vi "querey source settings menu small.vi"(0 "Enable":bool=TRUE, 1 "subvi?":bool, 5 "error in (no error)":errorcluster) -> (14 "Output cluster":T1={"Integer Timestamp"=0, "Needle Voltage"=0.0, "Frequency"=1.0, "Width (ms) : 0.1 "=0.05, "Desired Amplitude (V)"=0.0, "Settings ID"="", "ID#"=0} {"Needle Voltage" min=0.0 max=10.0 step=0.01 format="%.2g"; "Desired Amplitude (V)" min=0.0 max=10.0 step=0.01 format="%5.2f"; "Width (ms) : 0.1" min=0.05 max=5.0 step=0.01 format="%6.2f"; "Frequency" min=1.0 max=100.0 step=0.01 format="%.1f"}, 15 "Cancel loading":bool caption="Cancel", 18 "OK":bool, 19 "error out":errorcluster)   [LabVIEW 2012]
doc: "Displays a standard dialog box that prompts users to enter information, such as a user name and password.\n--------------------\n\nThis Express VI is configured as follows:\n\nMessage to Display to the User:\nThe inputs are: \nNumber: Upper Timestamp Range\nNumber: Lower Timestamp Range\nNumber: Settings ID"
uses:
  <vilib>/Utility/miscctls.llb/LVPointTypeDef.ctl
  <vilib>/addons/database/Auxilliary.llb/DB Tools Cursor Type.ctl
  <vilib>/addons/database/Connection.llb/Conn Execute.vi
  <vilib>/addons/database/Recordset.llb/Rec Fetch Recordset Data (R).vi
  <vilib>/addons/database/Recordset.llb/Rec Destroy - Connection.vi
  <vilib>/addons/database/_DB Variant To Data/Database Variant To Data.xnode
  <vilib>/addons/database/NI_Database_API.lvlib
panel:
  in  "Tag Filter":string
  out "Settings":cluster{"String":string, "Value":dbl}[](array[cluster])
  in  "Settings ID Type":enum32{"All", "Saved", "Big Accel", "Automatic"}(radio)
  in  "Needle Voltage":dbl
  in  "Frequency":dbl
  in  "Width (ms) : 0.1":dbl
  in  "Desired Amplitude (V)":dbl
  out "Settings to be loaded":string
  in  "OK2":bool
  in  "Cancel":bool
  in  "Settings ID":i32(ring) items=["Any Settings ID."=-1, "Big Accelerator: olivine (saved at  1/29/2014 1:59:55 PM)"=6, "olivine (saved at  1/29/2014 1:54:08 PM)"=5, "Big Accelerator: olivine (saved at  1/29/2014 1:53:03 PM)"=4, "test (saved at  1/29/2014 1:49:37 PM)"=3, "Big Accelerator: test (saved at  1/29/2014 1:49:28 PM)"=2, "0"=1]
  in  "Lower Timestamp Range":timestamp
  in  "Upper Timestamp Range":timestamp
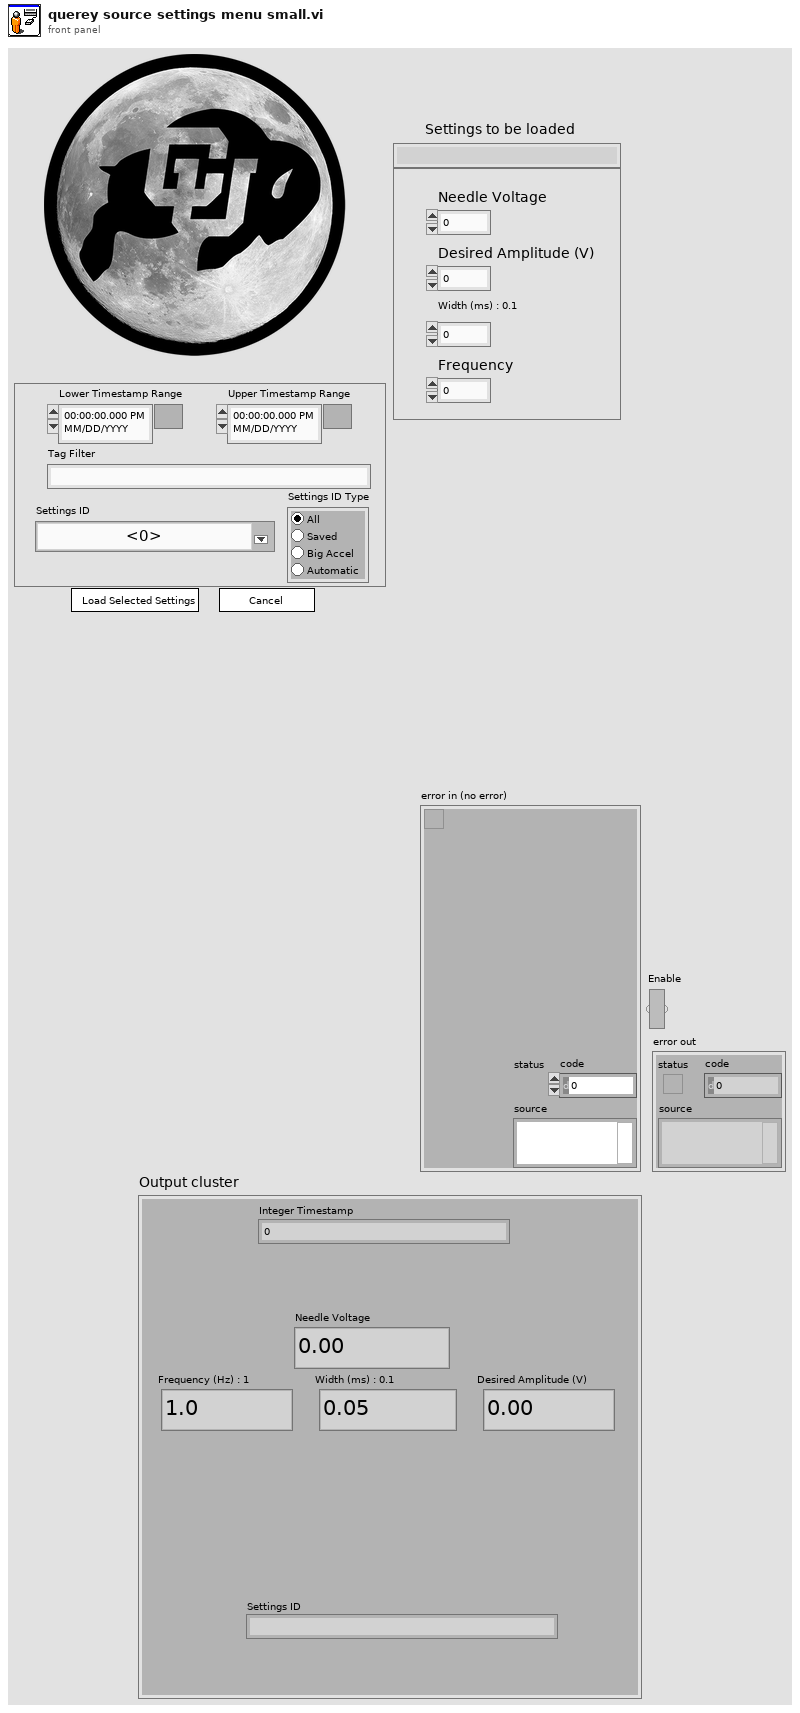
[diagram p1: front panel]
types:
  T1 = cluster{"Integer Timestamp":u64, "Needle Voltage":dbl, "Frequency":dbl, "Width (ms) : 0.1 ":dbl, "Desired Amplitude (V)":dbl, "Settings ID":string, "ID#":i32}
  T2 = typedef "LVPointTypeDef.ctl" = cluster{"Horizontal":i16, "Vertical":i16}
  T3 = enum32{"Invalid", "Standard", "Closed", "Hidden", "Minimized", "Maximized"}
  T4 = enum8{"Enabled", "Disabled", "Disabled and Grayed Out"}
  T5 = typedef "NI_Database_API.lvlib/DB Tools Cursor Type.ctl" = enum16{"forward-only", "keyset", "dynamic", "static"}
  T6 = typedef "NI_Database_API.lvlib/Conn ObjectReference.ctl" = refnum<k1>
  T7 = typedef "NI_Database_API.lvlib/Rec ObjectReference.ctl" = refnum<k1>
  T8 = typedef "dust_source_control_small.ctl" = cluster{"Integer Timestamp":u64, "Needle Voltage":dbl, "Frequency":dbl, "Width (ms) : 0.1 ":dbl, "Desired Amplitude (V)":dbl, "Settings ID":string, "ID#":i32}
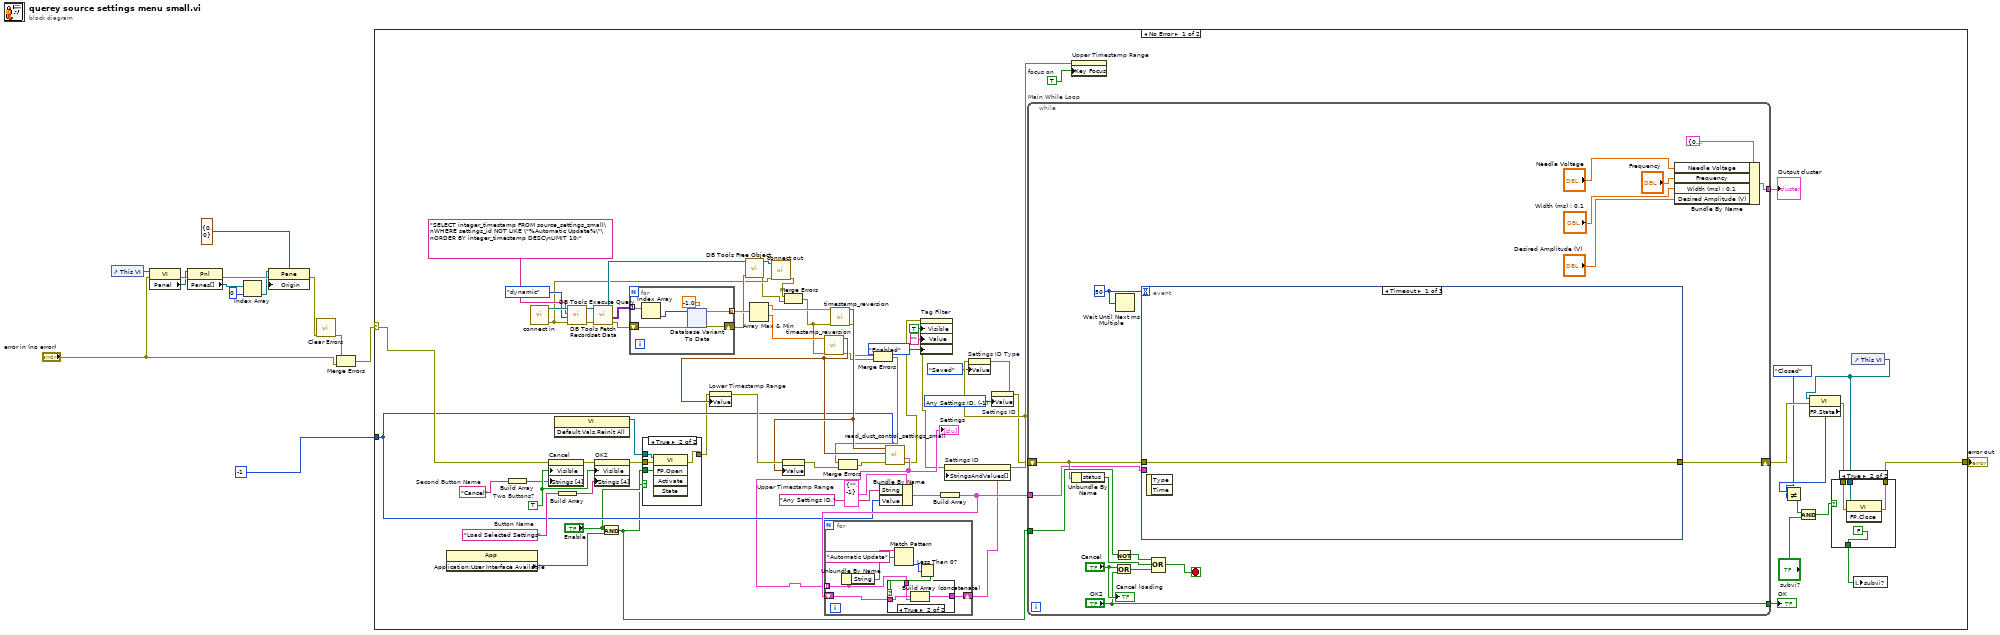
[diagram p0: block diagram]
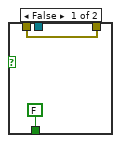
[diagram p2: hidden frame]
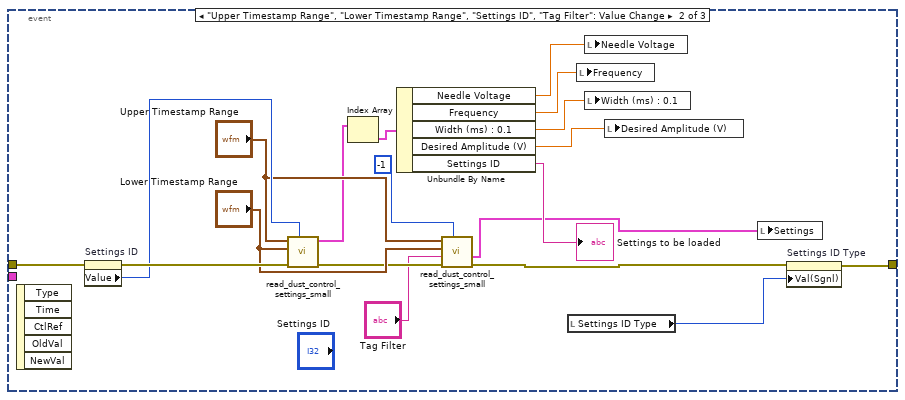
[diagram p5: hidden frame]
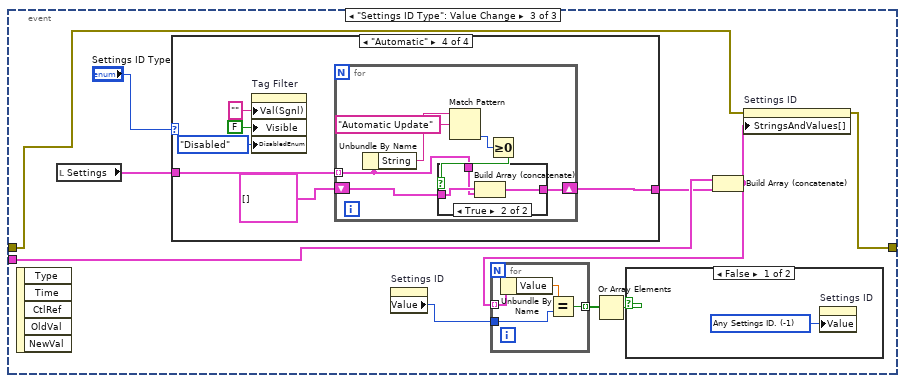
[diagram p6: hidden frame]
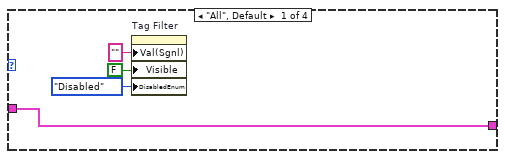
[diagram p8: hidden frame]
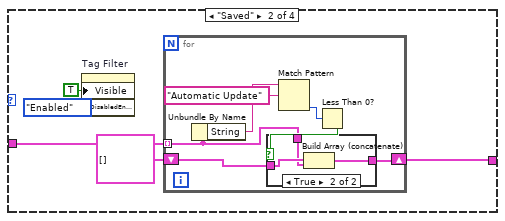
[diagram p9: hidden frame]
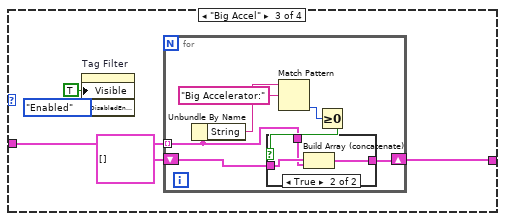
[diagram p11: hidden frame]
diagram:
  n1 = control-ref of="This VI"() -> (w12:refnum<vi>)
  n2 = property class="VI"(reference=w12, error in="error in (no error)") -> (error out=w11:errorcluster, "Panel"=w10:refnum<vi>)  [unwired: 1 out]
  n3 = property class="Pnl"(reference=w10, error in=w11) -> (error out=w9:errorcluster, "Panes[]"=w8:refnum<vi>[])  [unwired: 1 out]
  n4 = Index Array(array=w8, index=0) -> (element=w6:refnum<vi>)
  n5 = property class="Pane"(reference=w6, error in=w9, "Origin"=T2 {"Horizontal"=0, "Vertical"=0}) -> (error out=w4:errorcluster)  [unwired: 1 out]
  n6 = call <vilib>:"Clear Errors.vi"("error in (no error)"=w4) -> ("error out"=w2:errorcluster)  [unwired: 6 in]
  n7 = Merge Errors(w2, "error in (no error)") -> (w3:errorcluster)
  n8 = case shown="No Error" w3 {
    selector: w3 -> [w68 w248]
    tunnel: [w23 w248] -> w14
    tunnel: -1 ("Settings to be loaded") -> [w40 _]
    frame No Error {
      w35 = -1 items=["Any Settings ID."=-1, "Anna's Settings"=86, "Anna's Settings1"=87, "Test 'Test' \"Test\" test test."=97, "Test\""=91, "Test\""=92, "test 3"=82, "test 4"=83, "test mctesty"=88, "test mctesty"=89, "this is a \"test\" setting"=93] ("Settings ID")
      w74 = TRUE  # focus on
      w78 = "Cancel"  # Second Button Name
      w76 = "Load Selected Settings"  # Button Name
      w82 = TRUE  # Two Buttons?
      n9 = property class="App"() -> ("Application:User Interface Available"=w75:bool)  [unwired: 2 in, 2 out]
      n10 = Build Array(w78) -> (w79:string[])
      n11 = call "connect in.vi"() -> ("error out"=w52:errorcluster, "Database Connection"=w63:T6)  [unwired: 7 in, 1 out]
      n12 = property on="Cancel" class="Bool"(error in=w68, "Visible"=w82, "Strings [4]"=w79) -> (error out=w80:errorcluster)  [unwired: 1 in, 1 out]
      n13 = invoke class="VI" method="Default Vals.Reinit All"() -> (reference out=w29:refnum<vi>)  [unwired: 3 in, 2 out]
      n14 = Build Array(w76) -> (w77:string[])
      n15 = call-poly <vilib>:"DB Tools Execute Query.vi"("error in (no error)"=w52, "cursor type"=DB_Tools_Cursor_Type."dynamic", "SQL query"="SELECT integer_timestamp FROM source_settings_small\nWHERE settings_id NOT LIKE \"%Automatic Update%\"\nORDER BY integer_timestamp DESC\nLIMIT 10;" ("string"), "connection reference"=w63) -> ("error out"=w64:errorcluster, "recordset reference"=w65:T7)  [unwired: 4 in]
      n16 = call-poly <vilib>:"DB Tools Fetch Recordset Data.vi"("error in (no error)"=w64, "recordset reference"=w65) -> ("error out"=w59:errorcluster, "recordset data"=w60:variant[][], "recordset reference out"=w54:T7)  [unwired: 3 in]
      n17 = property on="OK2" class="Bool"(error in=w80, "Visible"=w82, "Strings [4]"=w77) -> (error out=w26:errorcluster)  [unwired: 1 in, 1 out]
      n18 = And(x="Enable", y=w75) -> (x .and. y?=w27:bool)
      n19 = for {
        tunnel: w60 -> [w109] mode=indexing
        tunnel: [w107] -> w58 mode=indexing
        shift-right: [w105] -> w53
        shift-left: w59 -> [w106]
        n20 = Index Array(array=w109) -> (element=w108:variant)  [unwired: 1 in]
        n21 = xnode "Database Variant To Data"("database variant"=w108, "error in (no error)"=w106, "type"=-1.0 ("Settings to be loaded")) -> ("data"=w107:dbl, "error out"=w105:errorcluster)
      }
      n22 = case shown="True" "Enable" {
        tunnel: w29 -> [_ w93]
        tunnel: w27 -> [_ w92]
        tunnel: w26 -> [w89 w91]
        tunnel: [w89 w90] -> w25
        frame False {
        }
        frame True {
          n23 = invoke class="VI" method="FP.Open"(reference=w93, error in=w91, "Activate"=w92) -> (error out=w90:errorcluster)  [unwired: 2 in, 4 out]
        }
      }
      n24 = call-poly <vilib>:"DB Tools Free Object.vi"("error in (no error)"=w53, "recordset reference"=w54) -> ("error out"=w51:errorcluster, "connection reference"=w55:T6)  [unwired: 8 in]
      n25 = Array Max & Min(array=w58) -> (max value=w57:dbl, min value=w56:dbl)  [unwired: 2 out]
      n26 = call "connect out.vi"("error in (no error)"=w52, "connection reference"=w55) -> ("error out"=w50:errorcluster)  [unwired: 9 in]
      n27 = Merge Errors(w50, w51) -> (w49:errorcluster)
      n28 = call "timestamp_reversion.vi"("error in (no error)"=w49, "Integer Timestamp"=w56) -> ("error out"=w45:errorcluster, "time stamp"=w47:timestamp)  [unwired: 7 in]
      n29 = property on="Lower Timestamp Range" class="AbsTime (strict)"(error in=w25, "Value"=w47) -> (error out=w72:errorcluster)  [unwired: 1 in, 1 out]
      n30 = call "timestamp_reversion.vi"("error in (no error)"=w49, "Integer Timestamp"=w57) -> ("error out"=w46:errorcluster, "time stamp"=w48:timestamp)  [unwired: 7 in]
      n31 = property on="Upper Timestamp Range" class="AbsTime (strict)"(error in=w72, "Value"=w48) -> (error out=w44:errorcluster)  [unwired: 1 in, 1 out]
      n32 = Merge Errors(w46, w45) -> (w43:errorcluster)
      n33 = Merge Errors(w43, w44) -> (w42:errorcluster)
      n34 = Bundle By Name(cluster=cluster{"String":string, "Value":i32} {"String"="", "Value"=-1}, "String"="Any Settings ID." ("Settings to be loaded"), "Value"=w40) -> (w69:cluster{"String":string, "Value":i32})
      n35 = call "read_dust_control_settings_small.vi"("Settings to be loaded"=w40, "error in (no error)"=w42, "Lower Timestamp Range"=w47, "Upper Timestamp Range"=w48) -> ("error out"=w32:errorcluster, "Array"=w38:cluster{"String":string, "Value":dbl}[])  [unwired: 5 in, 1 out]
      "Settings" <- w38
      n36 = property on="Tag Filter" class="Str"(error in=w32, "Visible"=TRUE, "Value"="" ("Tag"), "DisabledEnum"=T4."Enabled" ("Disabled")) -> (error out=w31:errorcluster)  [unwired: 1 in, 1 out]
      n37 = Build Array(w69) -> (w41:cluster{"String":string, "Value":i32}[])
      n38 = for {
        tunnel: w38 -> [w96] mode=indexing
        shift-right: [w95] -> w39
        shift-left: w41 -> [w97]
        n39 = Unbundle By Name(w96) -> ("String"=w100:string)
        n40 = Match Pattern(string=w100, regular expression="Automatic Update") -> (offset past match=w94:i32)  [unwired: 1 in, 3 out]
        n41 = Less Than 0?(x=w94) -> (x < 0?=w98:bool)
        n42 = case shown="True" w98 {
          tunnel: w97 -> [w101 w104]
          tunnel: w96 -> [_ w103]
          tunnel: [w101 w102] -> w95
          frame False {
          }
          frame True {
            n43 = Build Array (concatenate)(w104, w103) -> (w102:cluster{"String":string, "Value":dbl}[])
          }
        }
      }
      n44 = property on="Settings ID" class="Ring (strict)"(error in=w31, "StringsAndValues[]"=w39) -> (error out=w67:errorcluster)  [unwired: 1 in, 1 out]
      n45 = property on="Settings ID Type" class="RadioBtnsControl (strict)"(error in=w67, "Value"=enum32{"All", "Saved", "Big Accel", "Automatic"}."Saved" ("Settings ID Type")) -> (error out=w37:errorcluster)  [unwired: 1 in, 1 out]
      n46 = property on="Settings ID" class="Ring (strict)"(error in=w37, "Value"=w35) -> (error out=w36:errorcluster)  [unwired: 1 in, 1 out]
      n47 = while "Main While Loop" {
        tunnel: ["OK2"] -> w81
        tunnel: w27 -> [w158]
        tunnel: w41 -> [w143]
        tunnel: [w149] -> w73
        shift-right: [w151] -> w24
        shift-left: w36 -> [w152]
        stop <- w156 stop-if-true
        w150 = u32 50 ("millisecond multiple")
        n48 = Unbundle By Name(w152) -> ("status"=w154:bool)
        n49 = Or(x="Cancel", y="OK2") -> (x .or. y?=w155:bool)
        n50 = Not(x=w158) -> (.not. x?=w157:bool)
        n51 = Wait Until Next ms Multiple(millisecond multiple=w150) -> ()  [unwired: 1 out]
        n52 = event shown="[0] Timeout" {
          selector: _ -> [_ _ _]
          dyn-events: _ -> [_ _ _]
          timeout: w150 -> [_ _ _]
          tunnel: w152 -> [w160 w179 w187]
          tunnel: [w160 w165 w186] -> w151
          tunnel: w143 -> [_ _ w181]
          event Timeout {
            n53 = event-data() -> ()  [unwired: 1 in, 2 out]
          }
          event "Upper Timestamp Range", "Lower Timestamp Range", "Settings ID", "Tag Filter": Value Change {
            n54 = event-data() -> ()  [unwired: 1 in, 5 out]
            n55 = property on="Settings ID" class="Ring (strict)"(error in=w179) -> (error out=w178:errorcluster, "Value"=w177:i32)  [unwired: 1 in, 1 out]
            n56 = call "read_dust_control_settings_small.vi"("Settings to be loaded"=w177, "error in (no error)"=w178, "Lower Timestamp Range"="Lower Timestamp Range", "Upper Timestamp Range"="Upper Timestamp Range") -> ("error out"=w174:errorcluster, "Dust Source Array"=w161:T8[])  [unwired: 5 in, 1 out]
            n57 = Index Array(array=w161) -> (element=w162:T8)  [unwired: 1 in]
            n58 = Unbundle By Name(w162) -> ("Needle Voltage"=w173:dbl, "Frequency"=w172:dbl, "Width (ms) : 0.1"=w171:dbl, "Desired Amplitude (V)"=w170:dbl, "Settings ID"=→"Settings to be loaded":string)
            n59 = call "read_dust_control_settings_small.vi"("Settings to be loaded"=-1, "error in (no error)"=w174, "Tag"="Tag Filter", "Lower Timestamp Range"="Lower Timestamp Range", "Upper Timestamp Range"="Upper Timestamp Range") -> ("error out"=w166:errorcluster, "Array"=w164:cluster{"String":string, "Value":dbl}[])  [unwired: 4 in, 1 out]
            n60 = local read "Settings ID Type"() -> (w167:enum32{"All", "Saved", "Big Accel", "Automatic"})
            n61 = local write "Frequency"(w172) -> ()
            n62 = local write "Needle Voltage"(w173) -> ()
            n63 = local write "Width (ms) : 0.1"(w171) -> ()
            n64 = local write "Desired Amplitude (V)"(w170) -> ()
            n65 = local write "Settings"(w164) -> ()
            n66 = property on="Settings ID Type" class="RadioBtnsControl (strict)"(error in=w166, "Val(Sgnl)"=w167) -> (error out=w165:errorcluster)  [unwired: 1 in, 1 out]
          }
          event "Settings ID Type": Value Change {
            n67 = event-data() -> ()  [unwired: 1 in, 5 out]
            n68 = local read "Settings"() -> (w188:cluster{"String":string, "Value":dbl}[])
            n69 = case shown="\"Automatic\"" "Settings ID Type" {
              tunnel: w188 -> [w198 w203 w219 w236]
              tunnel: [w198 w201 w217 w235] -> w180
              frame "All", Default {
                n70 = property on="Tag Filter" class="Str"("Val(Sgnl)"="" ("Value (Signaling)"), "Visible"=FALSE, "DisabledEnum"=T4."Disabled" ("Disabled")) -> ()  [unwired: 2 in, 2 out]
              }
              frame "Saved" {
                n71 = property on="Tag Filter" class="Str"("Visible"=TRUE, "DisabledEnum"=T4."Enabled" ("Disabled")) -> ()  [unwired: 2 in, 2 out]
                n72 = for {
                  tunnel: w203 -> [w205] mode=indexing
                  shift-right: [w204] -> w201
                  shift-left: cluster{"String":string, "Value":i32}[] [] -> [w206]
                  n73 = Unbundle By Name(w205) -> ("String"=w210:string)
                  n74 = Match Pattern(string=w210, regular expression="Automatic Update") -> (offset past match=w208:i32)  [unwired: 1 in, 3 out]
                  n75 = Less Than 0?(x=w208) -> (x < 0?=w207:bool)
                  n76 = case shown="True" w207 {
                    tunnel: w206 -> [w211 w214]
                    tunnel: w205 -> [_ w213]
                    tunnel: [w211 w212] -> w204
                    frame False {
                    }
                    frame True {
                      n77 = Build Array (concatenate)(w214, w213) -> (w212:cluster{"String":string, "Value":dbl}[])
                    }
                  }
                }
              }
              frame "Big Accel" {
                n78 = property on="Tag Filter" class="Str"("Visible"=TRUE, "DisabledEnum"=T4."Enabled" ("Disabled")) -> ()  [unwired: 2 in, 2 out]
                n79 = for {
                  tunnel: w219 -> [w221] mode=indexing
                  shift-right: [w220] -> w217
                  shift-left: cluster{"String":string, "Value":i32}[] [] -> [w222]
                  n80 = Unbundle By Name(w221) -> ("String"=w226:string)
                  n81 = Match Pattern(string=w226, regular expression="Big Accelerator:") -> (offset past match=w224:i32)  [unwired: 1 in, 3 out]
                  n82 = Greater Or Equal To 0?(x=w224) -> (x >= 0?=w223:bool)
                  n83 = case shown="True" w223 {
                    tunnel: w222 -> [w227 w230]
                    tunnel: w221 -> [_ w229]
                    tunnel: [w227 w228] -> w220
                    frame False {
                    }
                    frame True {
                      n84 = Build Array (concatenate)(w230, w229) -> (w228:cluster{"String":string, "Value":dbl}[])
                    }
                  }
                }
              }
              frame "Automatic" {
                n85 = property on="Tag Filter" class="Str"("Val(Sgnl)"="" ("Value (Signaling)"), "Visible"=FALSE, "DisabledEnum"=T4."Disabled" ("Disabled")) -> ()  [unwired: 2 in, 2 out]
                n86 = for {
                  tunnel: w236 -> [w238] mode=indexing
                  shift-right: [w237] -> w235
                  shift-left: cluster{"String":string, "Value":i32}[] [] -> [w239]
                  n87 = Unbundle By Name(w238) -> ("String"=w243:string)
                  n88 = Match Pattern(string=w243, regular expression="Automatic Update") -> (offset past match=w241:i32)  [unwired: 1 in, 3 out]
                  n89 = Greater Or Equal To 0?(x=w241) -> (x >= 0?=w240:bool)
                  n90 = case shown="True" w240 {
                    tunnel: w239 -> [w244 w247]
                    tunnel: w238 -> [_ w246]
                    tunnel: [w244 w245] -> w237
                    frame False {
                    }
                    frame True {
                      n91 = Build Array (concatenate)(w247, w246) -> (w245:cluster{"String":string, "Value":dbl}[])
                    }
                  }
                }
              }
            }
            n92 = property on="Settings ID" class="Ring (strict)"() -> ("Value"=w185:i32)  [unwired: 2 in, 2 out]
            n93 = Build Array (concatenate)(w181, w180) -> (w182:cluster{"String":string, "Value":dbl}[])
            n94 = for {
              tunnel: w182 -> [w193] mode=indexing
              tunnel: w185 -> [w191]
              tunnel: [w190] -> w184 mode=indexing
              n95 = Unbundle By Name(w193) -> ("Value"=w192:dbl)
              n96 = Equal?(x=w192, y=w191) -> (x = y?=w190:bool)
            }
            n97 = Or Array Elements(Boolean array=w184) -> (logical OR=w183:bool)
            n98 = case shown="False" w183 {
              frame False {
                w194 = i16 -1 items=["Any Settings ID."=-1, "Anna's Settings"=86, "Anna's Settings1"=87, "Test 'Test' \"Test\" test test."=97, "Test\""=91, "Test\""=92, "test 3"=82, "test 4"=83, "test mctesty"=88, "test mctesty"=89, "this is a \"test\" setting"=93] ("Settings ID")
                n99 = property on="Settings ID" class="Ring (strict)"("Value"=w194) -> ()  [unwired: 2 in, 2 out]
              }
              frame True {
              }
            }
            n100 = property on="Settings ID" class="Ring (strict)"(error in=w187, "StringsAndValues[]"=w182) -> (error out=w186:errorcluster)  [unwired: 1 in, 1 out]
          }
        }
        n101 = Compound Arithmetic op=OR(w157, w154, w155) -> (w156:bool)
        n102 = Bundle By Name(cluster=T1 {"Integer Timestamp"=0, "Needle Voltage"=0.0, "Frequency"=1.0, "Width (ms) : 0.1 "=0.05, "Desired Amplitude (V)"=0.0, "Settings ID"="", "ID#"=0} ("Output cluster"), "Needle Voltage"="Needle Voltage", "Frequency"="Frequency", "Width (ms) : 0.1"="Width (ms) : 0.1", "Desired Amplitude (V)"="Desired Amplitude (V)") -> (w149:T1)
        "Cancel loading" <- "Cancel"
      }
      "OK" <- w81
      "Output cluster" <- w73
      n103 = property on="Upper Timestamp Range" class="AbsTime (strict)"(error in=w67, "Key Focus"=w74) -> ()  [unwired: 1 in, 2 out]
      n104 = control-ref of="This VI"() -> (w15:refnum<vi>)
      n105 = property class="VI"(reference=w15, error in=w24) -> (error out=w22:errorcluster, "FP.State"=w21:T3)  [unwired: 1 out]
      n106 = Not Equal?(x=w21, y=T3."Closed") -> (x != y?=w18:bool)
      n107 = And(x=w18, y="subvi?") -> (x .and. y?=w19:bool)
      n108 = case shown="True" w19 {
        tunnel: w22 -> [w84 w88]
        tunnel: [w84 w87] -> w23
        tunnel: [FALSE ("subvi?") FALSE ("subvi?")] -> w16
        tunnel: w15 -> [_ w85]
        frame False {
        }
        frame True {
          n109 = invoke class="VI" method="FP.Close"(reference=w85, error in=w88) -> (error out=w87:errorcluster)  [unwired: 1 in, 2 out]
        }
      }
      n110 = local write "subvi?"(w16) -> ()
    }
    frame Error {
    }
  }
  "error out" <- w14
